vi "Write Single Holding Register.vi"(8 "error in (no error)":errorcluster, 9 "holding register value":u16, 10 "address":u16, 11 "Modbus master in":refnum<class "Modbus Master.lvclass">) -> (0 "error out":errorcluster, 3 "Modbus master out":refnum<class "Modbus Master.lvclass">)   [LabVIEW 2021, in "Modbus Master.lvclass"]
doc: "Writes a value to a single holding register."
uses:
  Modbus Master.lvclass
  Modbus Master.lvclass/Modbus Master.ctl
  Modbus Data Unit/Modbus Data Unit.lvclass/Modbus Data Unit.ctl
  Network Protocol/Network Master/Network Master.lvclass/Network Master.ctl
  Master Function Definition/Write Single Register Request.vi
  Master Function Definition/Function data mismatch error.vi
  Master Function Definition/Write Single Register Response.vi
  Network Protocol/Network Master/Read write Master.vi
  Modbus Data Unit/Construct PDU.vi
  Master Function Definition/Function code mismatch error.vi
  Data Model/Error Generator.vi
  Modbus Data Unit/Deconstruct PDU.vi
  Modbus Data Unit/Modbus Data Unit.lvclass
  Transmission Data Unit/Transmission Data Unit.lvclass
  Network Protocol/Network Master/Network Master.lvclass
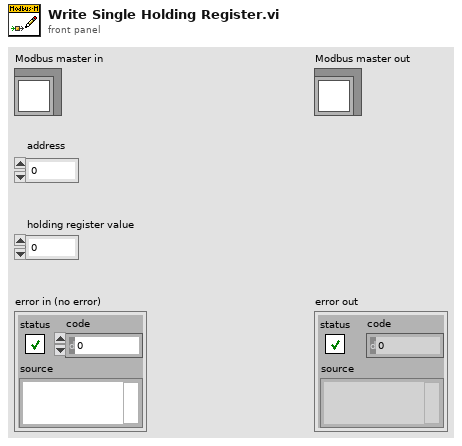
[diagram p1: front panel]
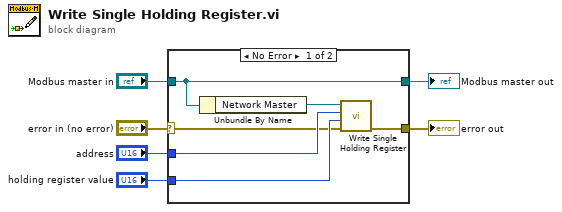
[diagram p0: block diagram]
diagram:
  n1 = case shown="No Error" "error in (no error)" {
    selector: "error in (no error)" -> [w7 w14]
    tunnel: "Modbus master in" -> [w8 w13]
    tunnel: [w8 w13] -> w4
    tunnel: [w12 w14] -> w3
    tunnel: "address" -> [w11 _]
    tunnel: "holding register value" -> [w10 _]
    frame No Error {
      n2 = Unbundle By Name(w8) -> ("Network Master"=w9:refnum<class "Network Master.lvclass">)
      n3 = call "Write Single Holding Register.vi"("error in (no error)"=w7, "holding register value"=w10, "address"=w11, "Modbus master in"=w9) -> ("error out"=w12:errorcluster)  [unwired: 6 in, 1 out]
    }
    frame Error {
    }
  }
  "error out" <- w3
  "Modbus master out" <- w4
